vi "set subject.vi"(8 "error in":errorcluster {"code" format="Error %.0f"}, 10 "subject":string, 11 "NATS Subscription in":refnum<class "NATS Subscription.lvclass">) -> (0 "error out":errorcluster {"code" format="Error %.0f"}, 3 "NATS Subscription out":refnum<class "NATS Subscription.lvclass">)   [LabVIEW 2020, in "NATS Subscription.lvlib" / "NATS Subscription.lvclass"]
uses:
  NATS Subscription.lvclass
  NATS Subscription.lvclass/NATS Subscription.ctl
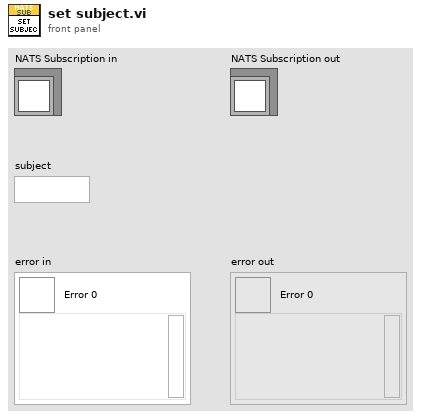
[diagram p1: front panel]
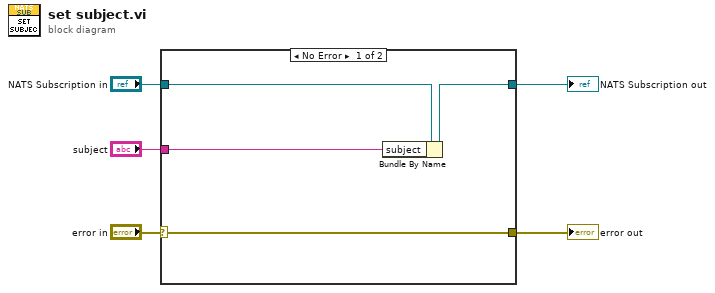
[diagram p0: block diagram]
diagram:
  n1 = case shown="No Error" "error in" {
    selector: "error in" -> [w9 w11]
    tunnel: [w9 w11] -> w4
    tunnel: [w7 w10] -> w2
    tunnel: "NATS Subscription in" -> [w8 w10]
    tunnel: "subject" -> [w6 _]
    frame No Error {
      n2 = Bundle By Name(cluster=w8, "subject"=w6) -> (w7:refnum<class "NATS Subscription.lvclass">)
    }
    frame Error {
    }
  }
  "error out" <- w4
  "NATS Subscription out" <- w2
